vi "control_daqmx_task.vi"(8 "error in":errorcluster, 9 "Test Section Physical Channels":T1={"Vapor Mass Flow Current"="cDAQ1Mod1/ai10", "Vapor Line Density Current"="cDAQ1Mod1/ai11", "Liquid Mass Flow Current"="cDAQ1Mod1/ai8", "Liquid Line Density Current"="cDAQ1Mod1/ai9", "Vapor Tank Pressure"="cDAQ1Mod1/ai3", "Liquid Tank Pressure"="cDAQ1Mod1/ai6", "Separator Pressure"="cDAQ1Mod1/ai2", "Liquid Inlet Pressure"="cDAQ1Mod1/ai4", "Vapor Inlet Pressure"="cDAQ1Mod1/ai0", "Vapor Tank Temperature"="cDAQ1Mod1/ai1", "Vapor Inlet Temperature"="cDAQ1Mod6/ai2", "Liquid Tank Temperature"="cDAQ1Mod6/ai0", "Liquid Inlet Temperature"="cDAQ1Mod6/ai3", "Separator Temperature"="cDAQ1Mod6/ai4", "Lower Dev Section Pressure"="cDAQ1Mod6/ai1", "Test Section Temperature"="cDAQ1Mod1/ai5", "Upper Dev Section Temperature"="cDAQ1Mod1/ai12", "Upper Dev Section Pressure"="cDAQ1Mod6/ai9", "Atmospheric Pressure"="cDAQ1Mod5/ai7", "Mixing Tee dP"="cDAQ1Mod6/ai5", "PG inlet-Mixing Tee Pressure"="cDAQ1Mod6/ai5", "Test Section Pressure"="cDAQ1Mod5/ai7"}) -> (0 "error out":errorcluster, 3 "task out":refnum<k21>)   [LabVIEW 2017]
uses:
  Input Channel Lists/test_section_physical_channels.ctl
  <vilib>/DAQmx/create/channels.llb/DAQmx Create Channel (AI-Current-Basic).vi
  <vilib>/DAQmx/create/channels.llb/DAQmx Create Channel (AI-Voltage-Basic).vi
  <vilib>/DAQmx/create/channels.llb/DAQmx Create Channel (AI-Temperature-Thermocouple).vi
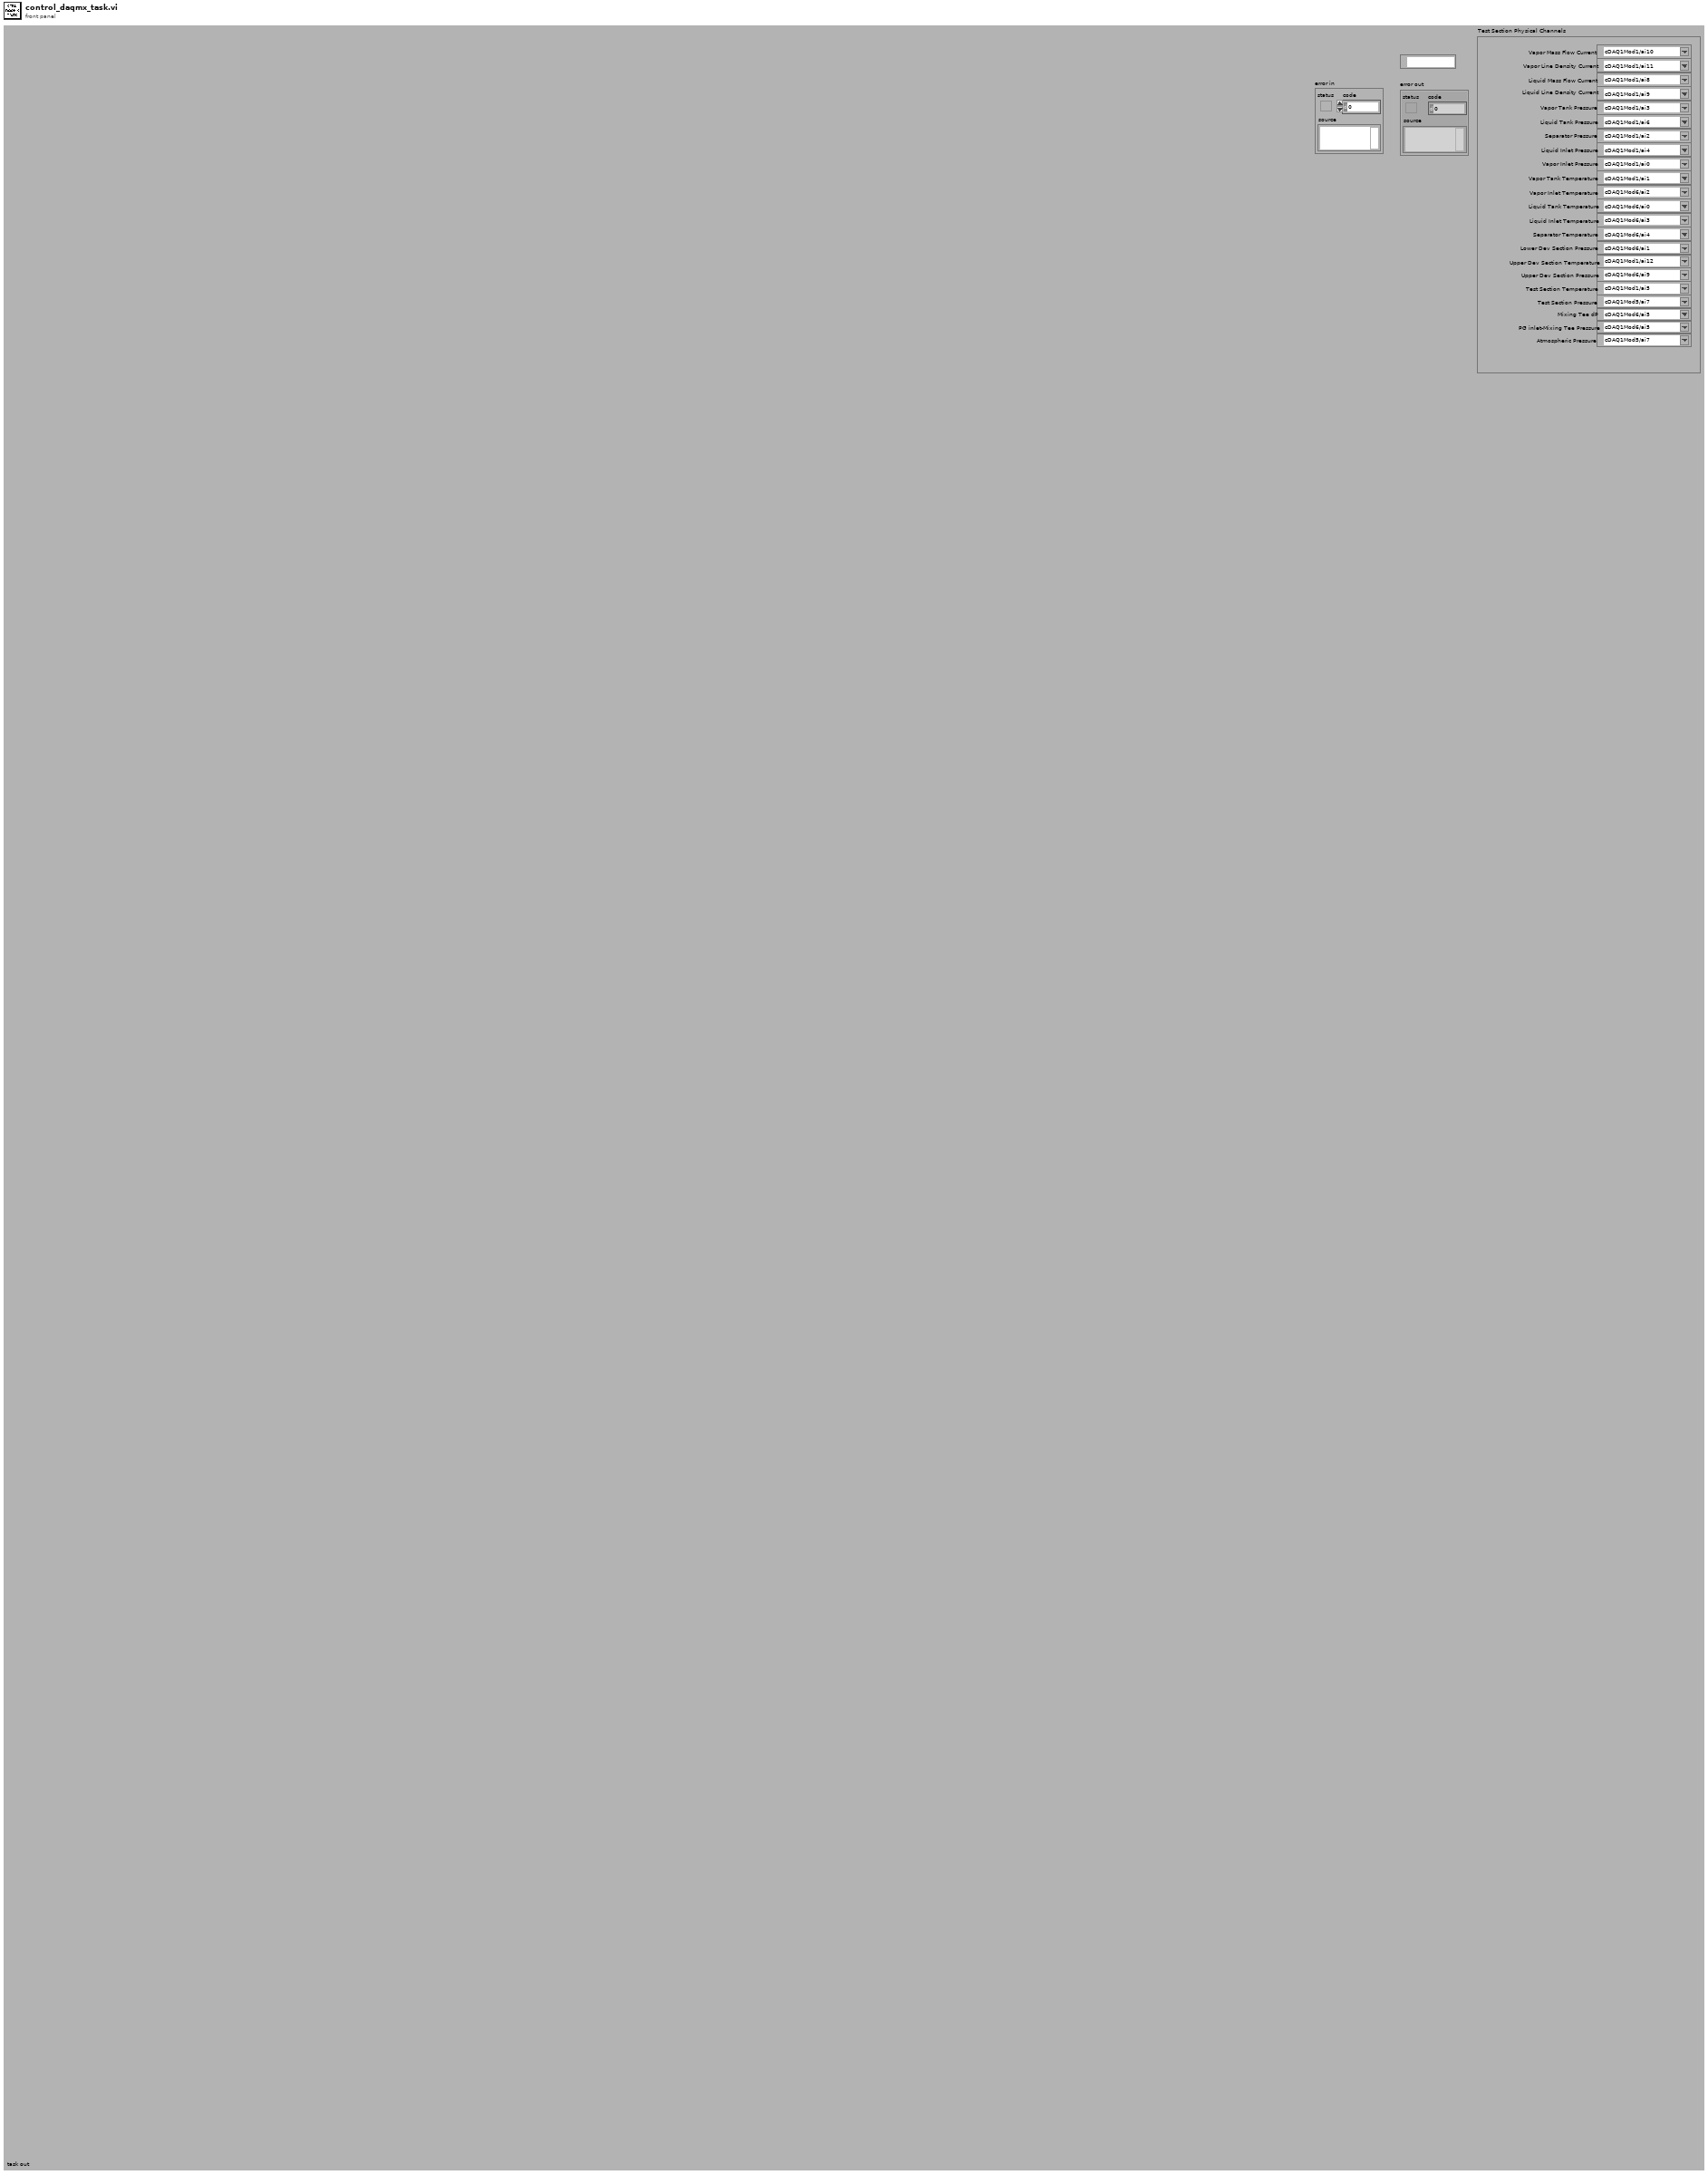
[diagram p1: front panel]
types:
  T1 = typedef "test_section_physical_channels.ctl" = cluster{"Vapor Mass Flow Current":tag, "Vapor Line Density Current":tag, "Liquid Mass Flow Current":tag, "Liquid Line Density Current":tag, "Vapor Tank Pressure":tag, "Liquid Tank Pressure":tag, "Separator Pressure":tag, "Liquid Inlet Pressure":tag, "Vapor Inlet Pressure":tag, "Vapor Tank Temperature":tag, "Vapor Inlet Temperature":tag, "Liquid Tank Temperature":tag, "Liquid Inlet Temperature":tag, "Separator Temperature":tag, "Lower Dev Section Pressure":tag, "Test Section Temperature":tag, "Upper Dev Section Temperature":tag, "Upper Dev Section Pressure":tag, "Atmospheric Pressure":tag, "Mixing Tee dP":tag, "PG inlet-Mixing Tee Pressure":tag, "Test Section Pressure":tag}
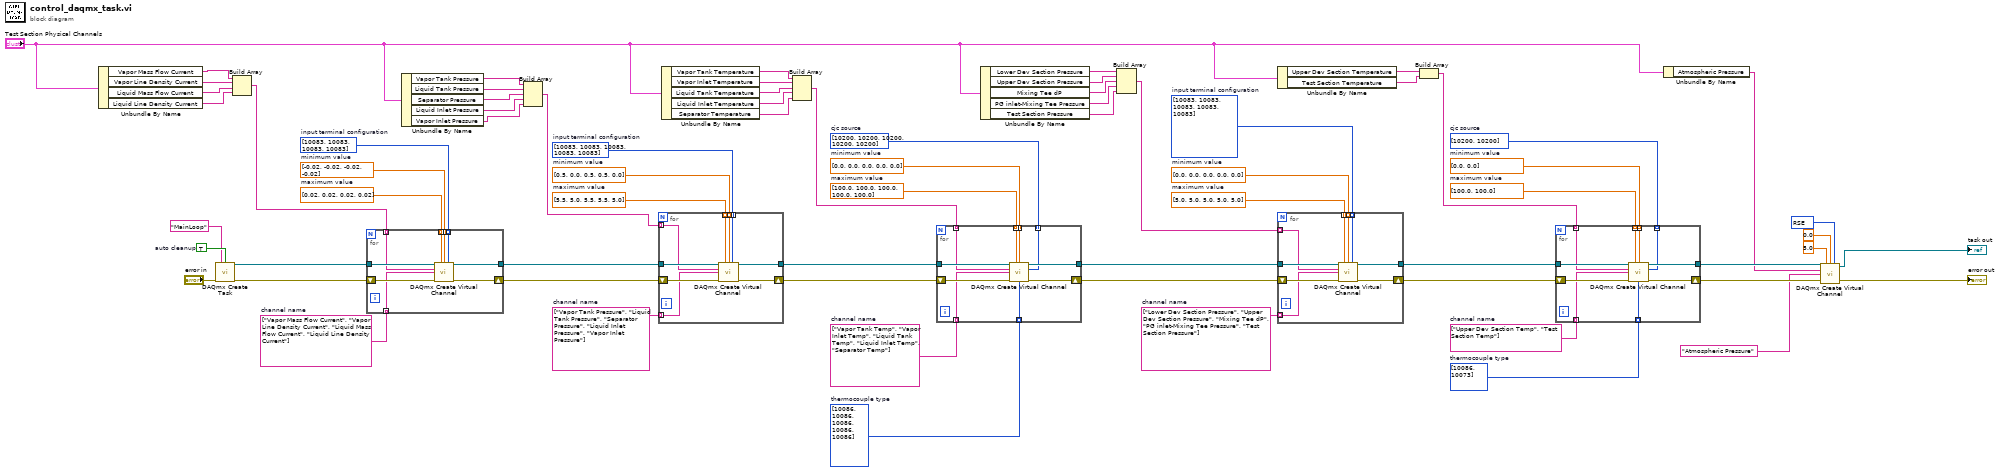
[diagram p0: block diagram]
diagram:
  w5 = 10083 items=["Default"=-1, "RSE"=10083, "NRSE"=10078, "Differential"=10106, "Pseudodifferential"=12529] ("input terminal configuration")
  w40 = i32[] [10086, 10073] items=["J"=10072, "K"=10073, "N"=10077, "R"=10082, "S"=10085, "T"=10086, "B"=10047, "E"=10055]  # thermocouple type
  w39 = string[] ["Upper Dev Section Temp", "Test Section Temp"]  # channel name
  w41 = dbl[] [100.0, 100.0]  # maximum value
  w42 = dbl[] [0.0, 0.0]  # minimum value
  w38 = u32[] [10200, 10200] items=["Internal"=10200, "Constant Value"=10116, "Channel"=10113]  # cjc source
  w45 = string[] ["Lower Dev Section Pressure", "Upper Dev Section Pressure", "Mixing Tee dP", "PG inlet-Mixing Tee Pressure", "Test Section Pressure"]  # channel name
  w46 = dbl[] [5.0, 5.0, 5.0, 5.0, 5.0]  # maximum value
  w47 = dbl[] [0.0, 0.0, 0.0, 0.0, 0.0]  # minimum value
  w48 = i32[] [10083, 10083, 10083, 10083, 10083] items=["default"=-1, "RSE"=10083, "NRSE"=10078, "Differential"=10106, "Pseudodifferential"=12529]  # input terminal configuration
  w53 = i32[] [10086, 10086, 10086, 10086, 10086] items=["J"=10072, "K"=10073, "N"=10077, "R"=10082, "S"=10085, "T"=10086, "B"=10047, "E"=10055]  # thermocouple type
  w52 = string[] ["Vapor Tank Temp", "Vapor Inlet Temp", "Liquid Tank Temp", "Liquid Inlet Temp", "Separator Temp"]  # channel name
  w54 = dbl[] [100.0, 100.0, 100.0, 100.0, 100.0]  # maximum value
  w55 = dbl[] [0.0, 0.0, 0.0, 0.0, 0.0]  # minimum value
  w50 = u32[] [10200, 10200, 10200, 10200, 10200] items=["Internal"=10200, "Constant Value"=10116, "Channel"=10113]  # cjc source
  w58 = string[] ["Vapor Tank Pressure", "Liquid Tank Pressure", "Separator Pressure", "Liquid Inlet Pressure", "Vapor Inlet Pressure"]  # channel name
  w59 = dbl[] [5.5, 5.0, 5.5, 5.5, 5.0]  # maximum value
  w60 = dbl[] [0.5, 0.0, 0.5, 0.5, 0.0]  # minimum value
  w61 = i32[] [10083, 10083, 10083, 10083, 10083] items=["default"=-1, "RSE"=10083, "NRSE"=10078, "Differential"=10106, "Pseudodifferential"=12529]  # input terminal configuration
  w64 = string[] ["Vapor Mass Flow Current", "Vapor Line Density Current", "Liquid Mass Flow Current", "Liquid Line Density Current"]  # channel name
  w65 = dbl[] [0.02, 0.02, 0.02, 0.02]  # maximum value
  w66 = dbl[] [-0.02, -0.02, -0.02, -0.02]  # minimum value
  w67 = i32[] [10083, 10083, 10083, 10083] items=["default"=-1, "RSE"=10083, "NRSE"=10078, "Differential"=10106, "Pseudodifferential"=12529]  # input terminal configuration
  w69 = TRUE  # auto cleanup
  n1 = Unbundle By Name("Test Section Physical Channels") -> ("Vapor Mass Flow Current"=w36:tag, "Vapor Line Density Current"=w35:tag, "Liquid Mass Flow Current"=w34:tag, "Liquid Line Density Current"=w33:tag)
  n2 = call <vilib>:"DAQmx Create Task.vi"("new task name"="MainLoop", "auto cleanup"=w69, "error in"="error in") -> ("task out"=w68:refnum<k21>, "error out"=w70:errorcluster)  [unwired: 11 in]
  n3 = Build Array(w36, w35, w34, w33) -> (w32:tag[])
  n4 = for {
    tunnel: w68 -> [w77]
    tunnel: w67 -> [w80] mode=indexing
    tunnel: w66 -> [w79] mode=indexing
    tunnel: w65 -> [w78] mode=indexing
    tunnel: w64 -> [w73] mode=indexing
    tunnel: w32 -> [w72] mode=indexing
    tunnel: [w75] -> w62
    shift-right: [w74] -> w63
    shift-left: w70 -> [w76]
    n5 = call-poly <vilib>:"DAQmx Create Virtual Channel.vi"("task in"=w77, "maximum value"=w78, "minimum value"=w79, "input terminal configuration"=w80, "physical channels"=w72, "name to assign"=w73, "error in"=w76) -> ("task out"=w75:refnum<k21>, "error out"=w74:errorcluster)  [unwired: 7 in]
  }
  n6 = Unbundle By Name("Test Section Physical Channels") -> ("Vapor Tank Pressure"=w28:tag, "Liquid Tank Pressure"=w29:tag, "Separator Pressure"=w30:tag, "Liquid Inlet Pressure"=w31:tag, "Vapor Inlet Pressure"=w22:tag)
  n7 = Build Array(w28, w29, w30, w31, w22) -> (w21:tag[])
  n8 = for {
    tunnel: w62 -> [w86]
    tunnel: w61 -> [w87] mode=indexing
    tunnel: w60 -> [w88] mode=indexing
    tunnel: w59 -> [w89] mode=indexing
    tunnel: w58 -> [w82] mode=indexing
    tunnel: w21 -> [w81] mode=indexing
    tunnel: [w84] -> w56
    shift-right: [w83] -> w57
    shift-left: w63 -> [w85]
    n9 = call-poly <vilib>:"DAQmx Create Virtual Channel.vi"("task in"=w86, "maximum value"=w89, "minimum value"=w88, "input terminal configuration"=w87, "physical channels"=w81, "name to assign"=w82, "error in"=w85) -> ("task out"=w84:refnum<k21>, "error out"=w83:errorcluster)  [unwired: 7 in]
  }
  n10 = Unbundle By Name("Test Section Physical Channels") -> ("Vapor Tank Temperature"=w27:tag, "Vapor Inlet Temperature"=w26:tag, "Liquid Tank Temperature"=w25:tag, "Liquid Inlet Temperature"=w24:tag, "Separator Temperature"=w20:tag)
  n11 = Build Array(w27, w26, w25, w24, w20) -> (w19:tag[])
  n12 = for {
    tunnel: w56 -> [w97]
    tunnel: w55 -> [w98] mode=indexing
    tunnel: w54 -> [w99] mode=indexing
    tunnel: w53 -> [w90] mode=indexing
    tunnel: w52 -> [w93] mode=indexing
    tunnel: w19 -> [w92] mode=indexing
    tunnel: [w95] -> w49
    tunnel: w50 -> [w91] mode=indexing
    shift-right: [w94] -> w51
    shift-left: w57 -> [w96]
    n13 = call-poly <vilib>:"DAQmx Create Virtual Channel.vi"("task in"=w97, "maximum value"=w99, "minimum value"=w98, "physical channels"=w92, "cjc source"=w91, "name to assign"=w93, "error in"=w96, "thermocouple type"=w90) -> ("task out"=w95:refnum<k21>, "error out"=w94:errorcluster)  [unwired: 6 in]
  }
  n14 = Unbundle By Name("Test Section Physical Channels") -> ("Lower Dev Section Pressure"=w23:tag, "Upper Dev Section Pressure"=w15:tag, "Mixing Tee dP"=w3:tag, "PG inlet-Mixing Tee Pressure"=w2:tag, "Test Section Pressure"=w1:tag)
  n15 = Build Array(w23, w15, w3, w2, w1) -> (w18:tag[])
  n16 = Unbundle By Name("Test Section Physical Channels") -> ("Upper Dev Section Temperature"=w17:tag, "Test Section Temperature"=w14:tag)
  n17 = for {
    tunnel: w49 -> [w105]
    tunnel: w48 -> [w106] mode=indexing
    tunnel: w47 -> [w107] mode=indexing
    tunnel: w46 -> [w108] mode=indexing
    tunnel: w45 -> [w101] mode=indexing
    tunnel: w18 -> [w100] mode=indexing
    tunnel: [w103] -> w43
    shift-right: [w102] -> w44
    shift-left: w51 -> [w104]
    n18 = call-poly <vilib>:"DAQmx Create Virtual Channel.vi"("task in"=w105, "maximum value"=w108, "minimum value"=w107, "input terminal configuration"=w106, "physical channels"=w100, "name to assign"=w101, "error in"=w104) -> ("task out"=w103:refnum<k21>, "error out"=w102:errorcluster)  [unwired: 7 in]
  }
  n19 = Build Array(w17, w14) -> (w16:tag[])
  n20 = for {
    tunnel: w43 -> [w116]
    tunnel: w42 -> [w117] mode=indexing
    tunnel: w41 -> [w118] mode=indexing
    tunnel: w40 -> [w109] mode=indexing
    tunnel: w39 -> [w112] mode=indexing
    tunnel: w16 -> [w111] mode=indexing
    tunnel: [w114] -> w13
    tunnel: w38 -> [w110] mode=indexing
    shift-right: [w113] -> w12
    shift-left: w44 -> [w115]
    n21 = call-poly <vilib>:"DAQmx Create Virtual Channel.vi"("task in"=w116, "maximum value"=w118, "minimum value"=w117, "physical channels"=w111, "cjc source"=w110, "name to assign"=w112, "error in"=w115, "thermocouple type"=w109) -> ("task out"=w114:refnum<k21>, "error out"=w113:errorcluster)  [unwired: 6 in]
  }
  n22 = Unbundle By Name("Test Section Physical Channels") -> ("Atmospheric Pressure"=w8:tag)
  n23 = call-poly <vilib>:"DAQmx Create Virtual Channel.vi"("task in"=w13, "maximum value"=5.0, "minimum value"=0.0, "input terminal configuration"=w5, "physical channels"=w8, "name to assign"="Atmospheric Pressure", "error in"=w12) -> ("task out"=→"task out":refnum<k21>, "error out"=→"error out":errorcluster)  [unwired: 7 in]
